vi "Exemple_Preprocessing_KBinsDiscretizer.vi"() -> ()   [LabVIEW 2020]
uses:
  Objet/6 - Datasets Transformation/6.3 - Processing Data/KBinsDiscretizer/KBinsDiscretizer.lvclass
panel:
  in  "Y":string[][](array[string])
  in  "X":string[][](array[string])=[["-2", "1", "-4", "-1"], ["-1", "2", "-3", "-0.5"], ["0", "3", "-2", "0.5"], ["1", "4", "-1", "2"]]
  out "Data":T1
  out "error out":errorcluster
  in  "error in":errorcluster caption="entrée d'erreur"
  in  "KBinsDiscretizer":T2={"n_bins"=[3], "encode"="ordinal", "strategy"="uniform"}
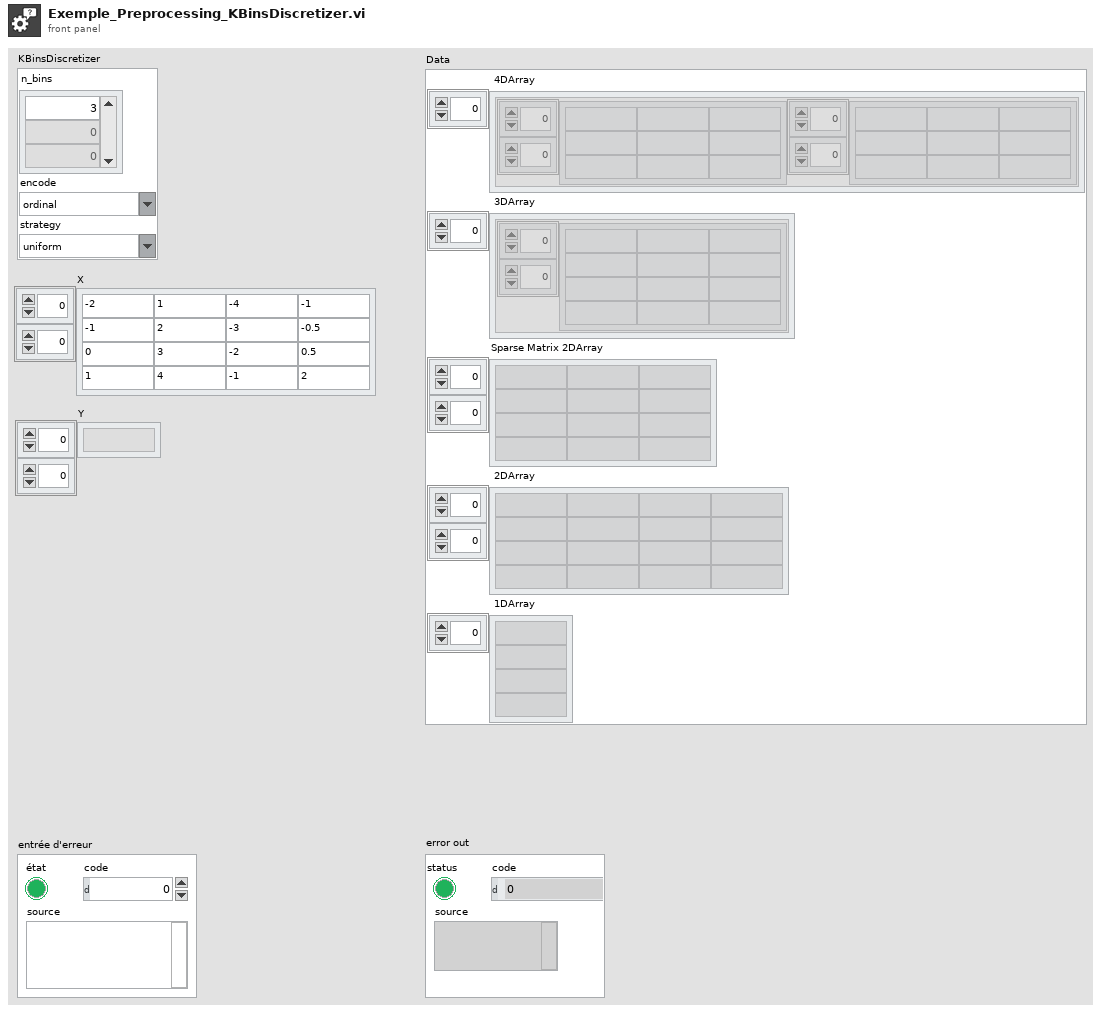
[diagram p1: front panel]
types:
  T1 = cluster{" 4DArray":cluster{"1":string[][], "2":string[][]}[], " 3DArray":cluster{"Tableau":string[][]}[], "Sparse Matrix 2DArray":string[][], " 2DArray":string[][], " 1DArray":string[]}
  T2 = cluster{"n_bins":i32[], "encode":string, "strategy":string}
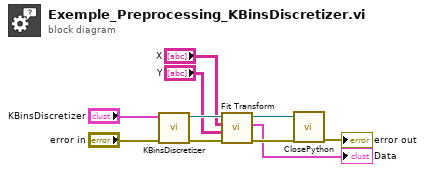
[diagram p0: block diagram]
diagram:
  n1 = call "KBinsDiscretizer.vi"("error in (no error)"="error in", "KBinsDiscretizer"="KBinsDiscretizer") -> ("error out"=w7:errorcluster, "KBinsDiscretizer.lvclass"=w8:refnum<class "KBinsDiscretizer.lvclass">)  [unwired: 8 in]
  n2 = call-dynamic "Fit Transform.vi"("error in (no error)"=w7, "y"="Y", "X"="X", "KBinsDiscretizer.lvclass"=w8) -> ("error out"=w6:errorcluster, "Data"=→"Data":T1, "KBinsDiscretizer.lvclass"=w5:refnum<class "KBinsDiscretizer.lvclass">)  [unwired: 5 in]
  n3 = call-dynamic "ClosePython.vi"("error in (no error)"=w6, "Scikit-learn en entrée"=w5) -> ("error out"=→"error out":errorcluster)  [unwired: 8 in, 1 out]
